vi "PWM.Measure.Digital.vi"(10 "State":bool, 11 "Channel.Settings":T3={"Active Edge"=FALSE, "Timeout Ticks"=1000000000}) -> (2 "Update?":bool, 3 "Cached.Data":T1)   [LabVIEW 2015]
uses:
  Types/PWM.Measure.Digital.Settings.ctl
  Types/PWM.Measure.Digital.Internal.ctl
  Types/PWM.Measure.Digital.Result.ctl
panel:
  out "Local.State":bool
  out "Local.Data":T2
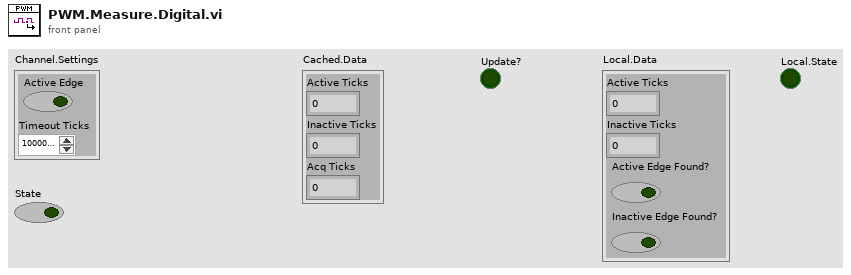
[diagram p1: front panel]
types:
  T1 = typedef "PWM.Measure.Digital.Result.ctl" = cluster{"Active Ticks":u32, "Inactive Ticks":u32, "Acq Ticks":u32}
  T2 = typedef "PWM.Measure.Digital.Internal.ctl" = cluster{"Active Ticks":u32, "Inactive Ticks":u32, "Active Edge Found?":bool, "Inactive Edge Found?":bool}
  T3 = typedef "PWM.Measure.Digital.Settings.ctl" = cluster{"Active Edge":bool, "Timeout Ticks":u32}
  T4 = enum8{"Initialize", "Wait on Active Edge", "Wait on Inactive Edge"}
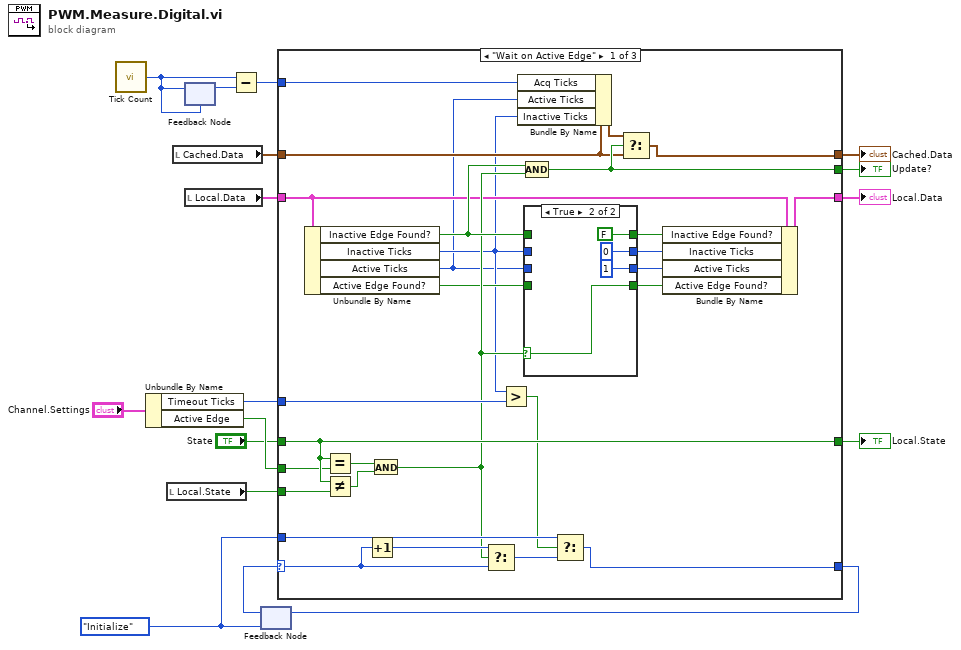
[diagram p0: block diagram]
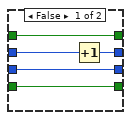
[diagram p2: hidden frame]
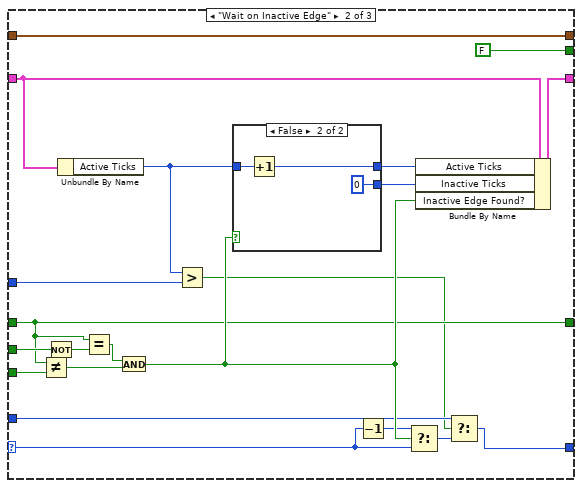
[diagram p3: hidden frame]
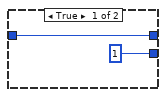
[diagram p4: hidden frame]
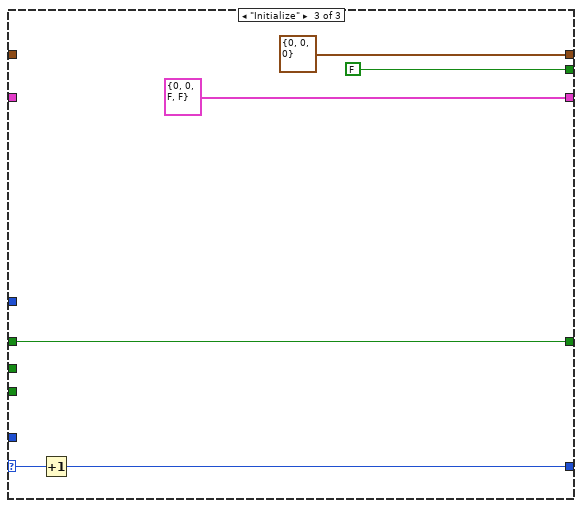
[diagram p5: hidden frame]
diagram:
  w7 = T4."Initialize"
  n1 = call "Tick Count"() -> ("Tick Count(Ticks)"=w3:u32)
  n2 = Unbundle By Name("Channel.Settings") -> ("Timeout Ticks"=w1:u32, "Active Edge"=w13:bool)
  n3 = local read "Local.State"() -> (w11:bool)
  n4 = local read "Cached.Data"() -> (w9:T1)
  n5 = feedback #1(w3) -> (w4:u32)
  n6 = feedback-in #1(w3) -> ()
  n7 = local read "Local.Data"() -> (w14:T2)
  n8 = Subtract(x=w3, y=w4) -> (x-y=w2:u32)
  n9 = feedback #2(w7) -> (w16:T4)
  n10 = case shown="\"Wait on Active Edge\"" w16 {
    selector: w16 -> [w44 w63 w86]
    tunnel: [w42 w73 T2 {"Active Ticks"=0, "Inactive Ticks"=0, "Active Edge Found?"=FALSE, "Inactive Edge Found?"=FALSE} ("Cached.Data")] -> w17
    tunnel: [w28 w56 w85] -> w15
    tunnel: w14 -> [w23 w72 _]
    tunnel: "State" -> [w37 w65 w84]
    tunnel: w13 -> [w35 w67 _]
    tunnel: [w37 w65 w84] -> w12
    tunnel: w11 -> [w45 w75 _]
    tunnel: [w38 w70 T1 {"Active Ticks"=0, "Inactive Ticks"=0, "Acq Ticks"=0} ("Cached.Data")] -> w10
    tunnel: w9 -> [w22 w70 _]
    tunnel: w1 -> [w32 w60 _]
    tunnel: w7 -> [w31 w59 _]
    tunnel: [w27 FALSE FALSE] -> w6
    tunnel: w2 -> [w19 _ _]
    frame "Wait on Active Edge" {
      n11 = Unbundle By Name(w23) -> ("Inactive Edge Found?"=w39:bool, "Inactive Ticks"=w20:u32, "Active Ticks"=w18:u32, "Active Edge Found?"=w24:bool)
      n12 = Equal?(x=w37, y=w35) -> (x = y?=w36:bool)
      n13 = Not Equal?(x=w37, y=w45) -> (x != y?=w34:bool)
      n14 = Increment(x=w44) -> (x+1=w43:T4)
      n15 = And(x=w36, y=w34) -> (x .and. y?=w26:bool)
      n16 = Select(t=w43, s=w26, f=w44) -> (s? t:f=w29:T4)
      n17 = Greater?(x=w20, y=w32) -> (0:w30:bool)
      n18 = Bundle By Name(cluster=w22, "Acq Ticks"=w19, "Active Ticks"=w18, "Inactive Ticks"=w20) -> (w21:T1)
      n19 = case shown="True" w26 {
        selector: w26 -> [_ w51]
        tunnel: [w49 u32 0 ("Inactive time")] -> w41
        tunnel: w20 -> [w50 _]
        tunnel: w39 -> [w48 _]
        tunnel: [w48 FALSE ("Inactive Edge Found?")] -> w40
        tunnel: [w47 u32 1 ("t")] -> w33
        tunnel: w18 -> [w47 _]
        tunnel: [w46 w51] -> w25
        tunnel: w24 -> [w46 _]
        frame False {
          n20 = Increment(x=w50) -> (x+1=w49:u32)
        }
        frame True {
        }
      }
      n21 = Compound Arithmetic op=AND(w39, w26) -> (w27:bool)
      n22 = Select(t=w31, s=w30, f=w29) -> (s? t:f=w28:T4)
      n23 = Select(t=w21, s=w27, f=w22) -> (s? t:f=w38:T1)
      n24 = Bundle By Name(cluster=w23, "Inactive Edge Found?"=w40, "Inactive Ticks"=w41, "Active Ticks"=w33, "Active Edge Found?"=w25) -> (w42:T2)
    }
    frame "Wait on Inactive Edge" {
      n25 = Not Equal?(x=w65, y=w75) -> (x != y?=w74:bool)
      n26 = Not(x=w67) -> (.not. x?=w66:bool)
      n27 = Unbundle By Name(w72) -> ("Active Ticks"=w61:u32)
      n28 = Equal?(x=w65, y=w66) -> (x = y?=w64:bool)
      n29 = And(x=w64, y=w74) -> (x .and. y?=w68:bool)
      n30 = Greater?(x=w61, y=w60) -> (0:w58:bool)
      n31 = case shown="False" w68 {
        tunnel: w61 -> [w77 w80]
        tunnel: [w77 w79] -> w71
        tunnel: [u32 1 ("t") u32 0 ("t")] -> w69
        frame True {
        }
        frame False {
          n32 = Increment(x=w80) -> (x+1=w79:u32)
        }
      }
      n33 = Decrement(x=w63) -> (x-1=w62:T4)
      n34 = Select(t=w62, s=w68, f=w63) -> (s? t:f=w57:T4)
      n35 = Bundle By Name(cluster=w72, "Active Ticks"=w71, "Inactive Ticks"=w69, "Inactive Edge Found?"=w68) -> (w73:T2)
      n36 = Select(t=w59, s=w58, f=w57) -> (s? t:f=w56:T4)
    }
    frame "Initialize" {
      n37 = Increment(x=w86) -> (x+1=w85:T4)
    }
  }
  "Local.Data" <- w17
  "Local.State" <- w12
  "Cached.Data" <- w10
  "Update?" <- w6
  n38 = feedback-in #2(w15) -> ()
